vi "Load Class Instance (parameter).vi"(7 "type":refnum<class>, 8 "error in":errorcluster, 9 "Search Folder":path, 10 "default library":string, 11 "parameter":string) -> (0 "error out":errorcluster, 3 "specific class reference":refnum<class>)   [LabVIEW 2021, in "Bananas.lvlib"]
uses:
  Bananas.lvlib
  <vilib>/LabVIEW Open Source Project/OpenURI/openURI.lvlib
  Class Search state -- enum.ctl
panel:
  out "state":T1=enum."Class not found"
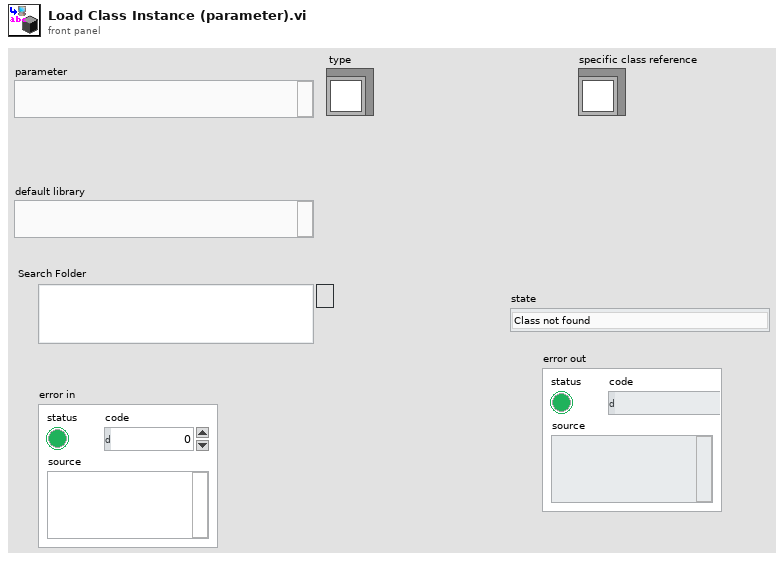
[diagram p1: front panel]
types:
  T1 = typedef "Bananas.lvlib/Class Search state -- enum.ctl" = enum16{"Fully Qualified Name in Memory", "Absolute Path", "Class Name, default lib in Memory", "Folder search", "Class not found", "Upstream Error"}
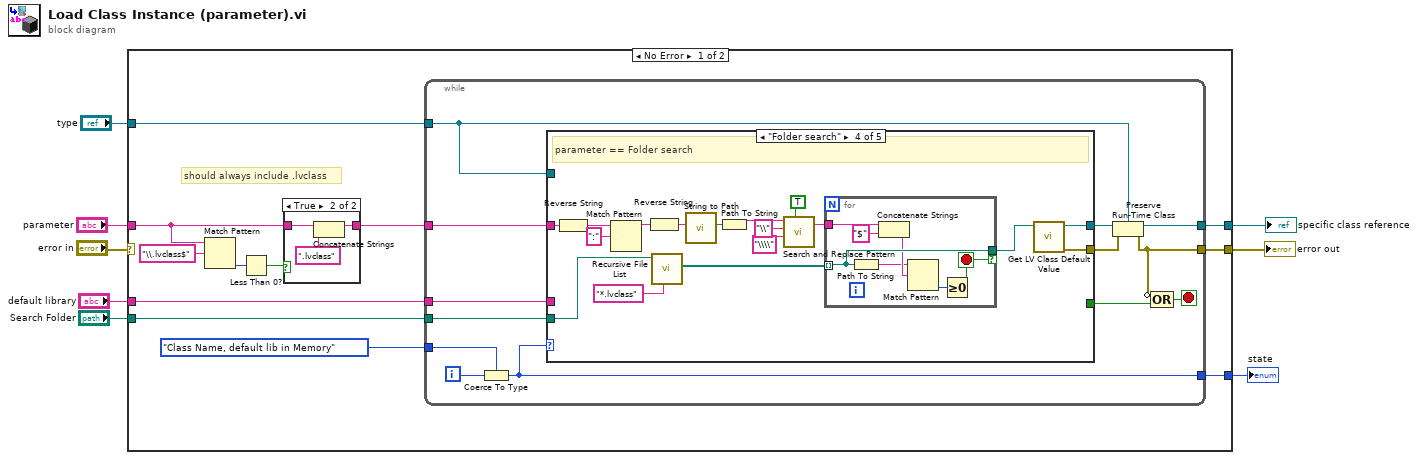
[diagram p0: block diagram]
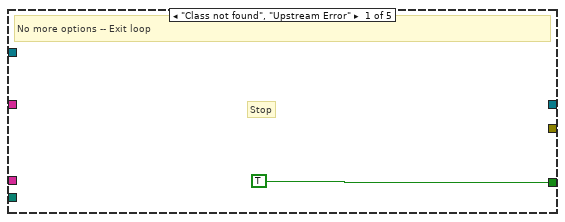
[diagram p3: hidden frame]
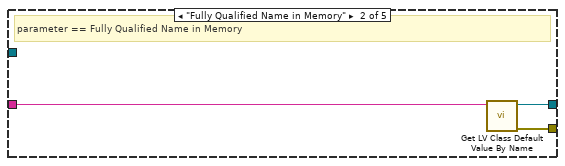
[diagram p4: hidden frame]
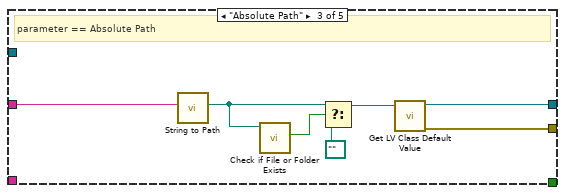
[diagram p5: hidden frame]
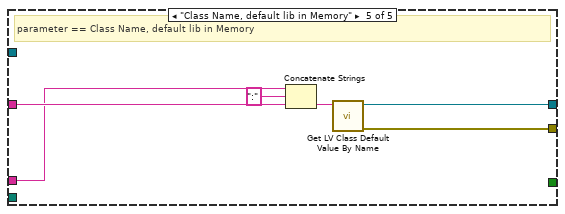
[diagram p6: hidden frame]
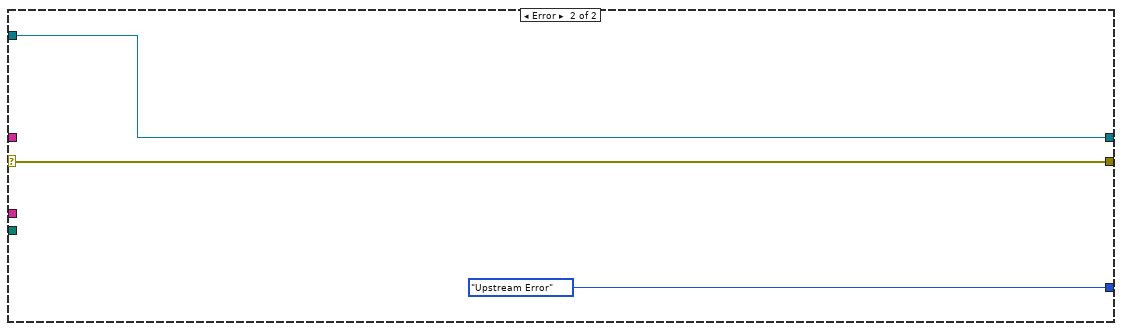
[diagram p7: hidden frame]
diagram:
  n1 = case shown="No Error" "error in" {
    selector: "error in" -> [_ w81]
    tunnel: [w20 w81] -> w8
    tunnel: [w19 w80] -> w7
    tunnel: "parameter" -> [w14 _]
    tunnel: "default library" -> [w12 _]
    tunnel: "Search Folder" -> [w11 _]
    tunnel: [w10 Class_Search_state_--_enum."Upstream Error"] -> w3
    tunnel: "type" -> [w9 w80]
    frame No Error {
      # "should always include .lvclass"
      n2 = Match Pattern(string=w14, regular expression="\\.lvclass$") -> (offset past match=w16:i32)  [unwired: 1 in, 3 out]
      n3 = Less Than 0?(x=w16) -> (x < 0?=w17:bool)
      n4 = case shown="True" w17 {
        tunnel: [w21 w23] -> w13
        tunnel: w14 -> [w21 w22]
        frame False {
        }
        frame True {
          n5 = Concatenate Strings(w22, ".lvclass" ("regular expression")) -> (w23:string)
        }
      }
      n6 = while {
        tunnel: w13 -> [w35]
        tunnel: [w32] -> w20
        tunnel: [w34] -> w19
        tunnel: w9 -> [w33]
        tunnel: Class_Search_state_--_enum."Class Name, default lib in Memory" -> [w29]
        tunnel: [w27] -> w10
        tunnel: w12 -> [w26]
        tunnel: w11 -> [w25]
        i -> [w28]
        stop <- w31 stop-if-true
        n7 = Coerce To Type(0:w28, 1:w29) -> (2:w27:T1)
        n8 = case shown="\"Folder search\"" w27 {
          tunnel: [_ w41 w48 w65 w78] -> w37
          tunnel: [_ w40 w47 w64 w77] -> w36
          tunnel: w35 -> [_ w39 w46 w63 w76]
          tunnel: w33 -> [_ _ _ _ _]
          tunnel: [TRUE _ _ _ _] -> w30
          tunnel: w26 -> [_ _ _ _ w75]
          tunnel: w25 -> [_ _ _ w58 _]
          frame "Class not found", "Upstream Error" {
            # "Stop"
            # "No more options -- Exit loop"
          }
          frame "Fully Qualified Name in Memory" {
            # "parameter == Fully Qualified Name in Memory"
            n9 = call <vilib>:"Get LV Class Default Value By Name.vi"("class name"=w39) -> ("error out"=w40:errorcluster, "object"=w41:refnum<class>)  [unwired: 9 in]
          }
          frame "Absolute Path" {
            # "parameter == Absolute Path"
            n10 = call <vilib>:"String to Path.vi"("common path"=w46) -> ("Path"=w44:path)  [unwired: 10 in]
            n11 = call <vilib>:"Check if File or Folder Exists.vi"("path"=w44) -> ("file or folder exists?"=w45:bool)  [unwired: 8 in, 2 out]
            n12 = Select(t=w44, s=w45, f=path "") -> (s? t:f=w43:path)
            n13 = call <vilib>:"Get LV Class Default Value.vi"("class path"=w43) -> ("error out"=w47:errorcluster, "object"=w48:refnum<class>)  [unwired: 9 in]
          }
          frame "Folder search" {
            # "parameter == Folder search"
            n14 = Reverse String(1:w63) -> (0:w61:string)
            n15 = Match Pattern(string=w61, regular expression=":") -> (before substring=w60:string)  [unwired: 1 in, 3 out]
            n16 = Reverse String(1:w60) -> (0:w59:string)
            n17 = call <vilib>:"Recursive File List.vi"("pattern"="*.lvclass", "Folder Path"=w58) -> ("All Files in Dir"=w56:path[])  [unwired: 5 in, 4 out]
            n18 = call <vilib>:"String to Path.vi"("common path"=w59) -> ("Path"=w55:path)  [unwired: 10 in]
            n19 = Path To String(path=w55) -> (string=w49:string)
            n20 = call <vilib>:"Search and Replace Pattern.vi"("string"=w49, "regular expression (\"\")"="\\" ("regular expression (\"\")"), "replace string (\"\")"="\\\\" ("regular expression (\"\")"), "replace all? (F)"=TRUE) -> ("result string"=w51:string)  [unwired: 1 in, 1 out]
            n21 = for {
              tunnel: w56 -> [w69] mode=indexing
              tunnel: w51 -> [w72]
              tunnel: [w69] -> w54 if=w68
              stop <- w68 stop-if-true
              n22 = Path To String(path=w69) -> (string=w66:string)
              n23 = Concatenate Strings(w72, "$" ("string")) -> (w67:string)
              n24 = Match Pattern(string=w66, regular expression=w67) -> (offset past match=w70:i32)  [unwired: 1 in, 3 out]
              n25 = Greater Or Equal To 0?(x=w70) -> (x >= 0?=w68:bool)
            }
            n26 = call <vilib>:"Get LV Class Default Value.vi"("class path"=w54) -> ("error out"=w64:errorcluster, "object"=w65:refnum<class>)  [unwired: 9 in]
          }
          frame "Class Name, default lib in Memory" {
            # "parameter == Class Name, default lib in Memory"
            n27 = Concatenate Strings(w75, ":" ("string"), w76) -> (w73:string)
            n28 = call <vilib>:"Get LV Class Default Value By Name.vi"("class name"=w73) -> ("error out"=w77:errorcluster, "object"=w78:refnum<class>)  [unwired: 9 in]
          }
        }
        n29 = Preserve Run-Time Class(object in=w37, error in=w36, 2:w33) -> (object out=w34:refnum<class>, error out=w32:errorcluster)
        n30 = Compound Arithmetic op=OR(invert w32, w30) -> (w31:bool)
      }
    }
    frame Error {
    }
  }
  "error out" <- w8
  "specific class reference" <- w7
  "state" <- w3
